vi "SetBitfiledValue(I64).vi"(8 "error in (no error)":errorcluster, 9 "bitfield value":i64, 10 "bitfield caps":T1={"offset"=0, "size"=0, "signed?"=TRUE}, 11 "original value":u64 format="%.0x") -> (0 "error out":errorcluster, 3 "update value":u64 format="%.0x")   [LabVIEW 2017, in "Bitfield.lvlib"]
uses:
  Bitfield.lvlib
  BitfieldCaps.ctl
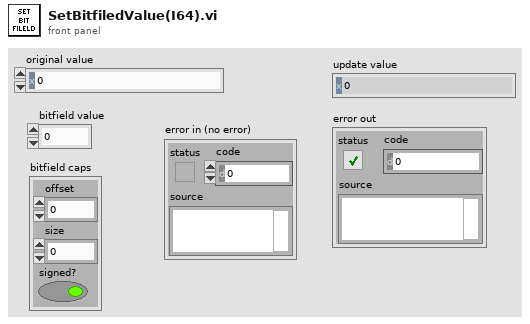
[diagram p1: front panel]
types:
  T1 = typedef "Bitfield.lvlib/BitfieldCaps.ctl" = cluster{"offset":i32, "size":i32, "signed?":bool}
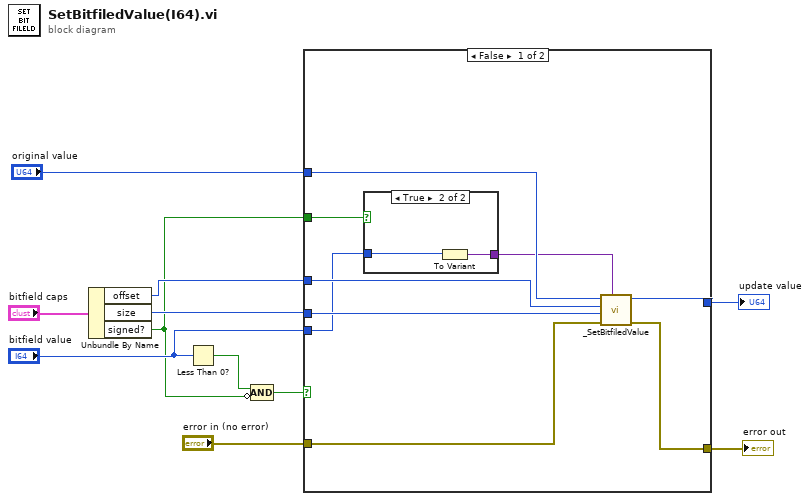
[diagram p0: block diagram]
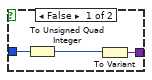
[diagram p2: hidden frame]
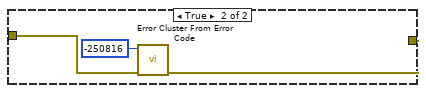
[diagram p3: hidden frame]
diagram:
  n1 = Unbundle By Name("bitfield caps") -> ("offset"=w3:i32, "size"=w2:i32, "signed?"=w1:bool)
  n2 = Less Than 0?(x="bitfield value") -> (x < 0?=w11:bool)
  n3 = Compound Arithmetic op=AND(w11, invert w1) -> (w10:bool)
  n4 = case shown="False" w10 {
    tunnel: "error in (no error)" -> [w20 w28]
    tunnel: [w18 w26] -> w5
    tunnel: w3 -> [w19 _]
    tunnel: w2 -> [w15 _]
    tunnel: "bitfield value" -> [w12 _]
    tunnel: "original value" -> [w17 _]
    tunnel: [w16 _] -> w6
    tunnel: w1 -> [w13 _]
    frame False {
      n5 = case shown="True" w13 {
        tunnel: [w23 w25] -> w14
        tunnel: w12 -> [w22 w24]
        frame False {
          n6 = To Unsigned Quad Integer(1:w22) -> (0:w21:u64)
          n7 = To Variant(anything=w21) -> (Variant=w23:variant)
        }
        frame True {
          n8 = To Variant(anything=w24) -> (Variant=w25:variant)
        }
      }
      n9 = call "_SetBitfiledValue.vi"("bitfield value"=w14, "error in (no error)"=w20, "size"=w15, "offset"=w19, "soft value"=w17) -> ("error out"=w18:errorcluster, "update value"=w16:u64)  [unwired: 4 in, 1 out]
    }
    frame True {
      n10 = call <vilib>:"Error Cluster From Error Code.vi"("error in (no error)"=w28, "error code (0)"=-250816) -> ("error out"=w26:errorcluster)  [unwired: 7 in]
    }
  }
  "update value" <- w6
  "error out" <- w5
